vi "DUAL GAUGE-Serial Init.vi"(8 "error in (no error)":errorcluster caption="Fehler (Eingang)", 10 "Baud Rate":u16(ring)=5 items=["300", "1200", "2400", "4800", "9600", "19200"], 11 "input refnum":refnum<visa-resource-name> caption="Eingang (Referenz)") -> (0 "error out":errorcluster caption="Fehler (Ausgang)", 3 "VISA resource out":refnum<visa-resource-name>)   [LabVIEW 2017, in "Dual Gauge.lvlib"]
uses:
  <userlib>/Dual Gauge/Dual Gauge.lvlib
  <vilib>/Instr/_visa.llb/VISA Configure Serial Port (Instr).vi
panel:
  in  "Baud Rate":u16[](array[numeric])=[300, 1200, 2400, 4800, 9600, 19200, 38400]
  in  "Buffer":u16=5000
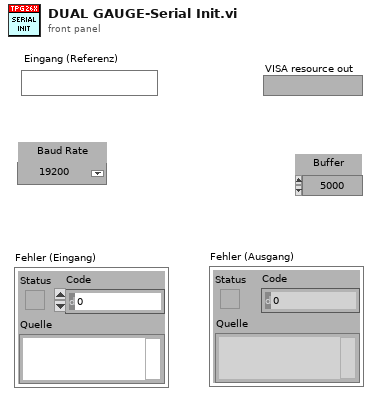
[diagram p1: front panel]
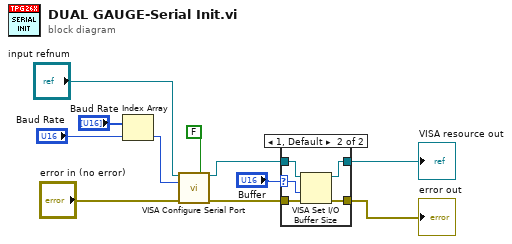
[diagram p0: block diagram]
diagram:
  n1 = Index Array(array="Baud Rate", index="Baud Rate") -> (element=w8:u16)
  n2 = call-poly "VISA Configure Serial Port"("VISA resource name"="input refnum", "Enable Termination\nChar (T)"=FALSE ("Enable Termination\nChar (T)"), "baud rate (9600)"=w8, "error in (no error)"="error in (no error)") -> ("VISA resource name out"=w4:refnum<visa-resource-name>, "error out"=w3:errorcluster)  [unwired: 10 in]
  n3 = case shown="1, Default" "Buffer" {
    selector: "Buffer" -> [_ w17]
    tunnel: w4 -> [w12 w18]
    tunnel: w3 -> [w13 w16]
    tunnel: [w13 w15] -> w1
    tunnel: [w12 w14] -> w5
    frame 0 {
    }
    frame 1, Default {
      n4 = VISA Set I/O Buffer Size(VISA resource name=w18, size (4096)=w17, error in (no error)=w16) -> (VISA resource name out=w14:refnum<visa-resource-name>, error out=w15:errorcluster)  [unwired: 1 in]
    }
  }
  "VISA resource out" <- w5
  "error out" <- w1
